vi "acquireValue.vi"(8 "error in (no error)":errorcluster, 10 "nextSample?":bool, 11 "startScan in":refnum<class "startScan.lvclass">) -> (0 "error out":errorcluster, 1 "function return":i32, 2 "variantData":variant, 3 "startScan out":refnum<class "startScan.lvclass">)   [LabVIEW 2016, in "SALLV_MtAtElectrometer_Messaging.lvlib" / "startScan.lvclass"]
uses:
  startScan.lvclass
  ts_sallv_MtAtElectrometer/SALLV_MtAtElectrometer.lvlib
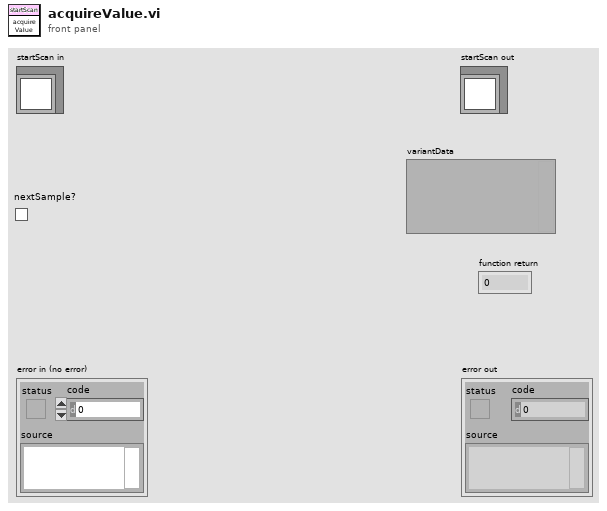
[diagram p1: front panel]
types:
  T1 = typedef "SALLV_MtAtElectrometer.lvlib/command_startScan.ctl" = cluster{"value":bool}
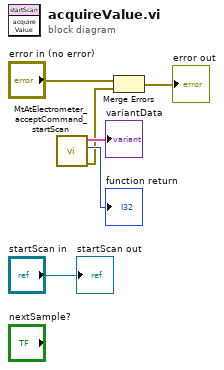
[diagram p0: block diagram]
diagram:
  n1 = call "MtAtElectrometer_acceptCommand_startScan.vi"() -> ("error out"=w1:errorcluster, "function return"=→"function return":i32, "command_startScan_Ctl out"=→"variantData":T1)  [unwired: 9 in]
  n2 = Merge Errors("error in (no error)", w1) -> (→"error out":errorcluster)
  "startScan out" <- "startScan in"
